vi "Deinitialize Robot.vi"(8 "error in":errorcluster, 11 "Gantry in":refnum<class "Gantry.lvclass">) -> (0 "error out":errorcluster, 3 "Gantry out":refnum<class "Gantry.lvclass">)   [LabVIEW 2026, in "Gantry.lvclass"]
uses:
  Gantry.lvclass
  <instrlib>/Aerotech Automation1/Aerotech Automation1.lvlib
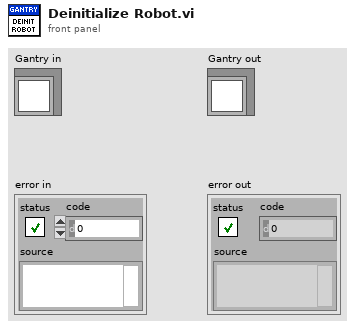
[diagram p1: front panel]
types:
  T1 = typedef "Virtual Modes.ctl" = enum16{"Nonvirtual", "Virtual"}
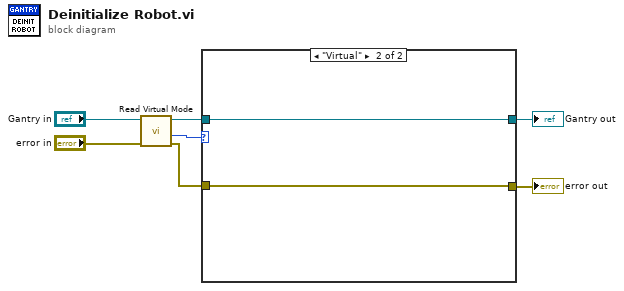
[diagram p0: block diagram]
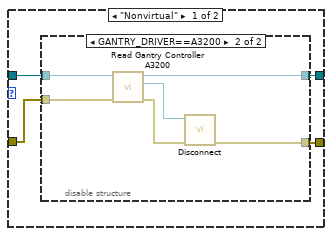
[diagram p2: hidden frame]
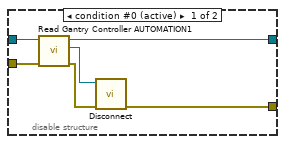
[diagram p3: hidden frame]
diagram:
  n1 = call-dynamic "Read Virtual Mode.vi"("error in (no error)"="error in", "Gantry in"="Gantry in") -> ("error out"=w3:errorcluster, "Virtual Mode"=w2:T1, "Gantry out"=w5:refnum<class "Gantry.lvclass">)  [unwired: 6 in, 1 out]
  n2 = case shown="\"Virtual\"" w2 {
    tunnel: [w9 w24] -> w7
    tunnel: w3 -> [w10 w24]
    tunnel: w5 -> [w11 w25]
    tunnel: [w8 w25] -> w1
    frame "Nonvirtual" {
      n3 = disable-structure shown="GANTRY_DRIVER==A3200" {
        disable-tunnel: w11 -> [w17 w21]
        disable-tunnel: w10 -> [w16 w20]
        disable-tunnel: [w13 w19] -> w9
        disable-tunnel: [w12 w18] -> w8
        frame condition #0 (active) {
          n4 = call "Read Gantry Controller AUTOMATION1.vi"("error in (no error)"=w16, "Gantry in"=w17) -> ("error out"=w15:errorcluster, "Controller AUTOMATION1"=w14:refnum<k24>, "Gantry out"=w12:refnum<class "Gantry.lvclass">)  [unwired: 7 in]
          n5 = call <instrlib>:"Disconnect.vi"("error in (no error)"=w15, "Controller Refnum in"=w14) -> ("error out"=w13:errorcluster)  [unwired: 9 in]
        }
        frame condition #1 {
          n6 = call "Read Gantry Controller A3200.vi"("error in (no error)"=w20, "Gantry in"=w21) -> ("error out"=w23:errorcluster, "A3200 controller out"=w22:refnum<k24>, "Gantry out"=w18:refnum<class "Gantry.lvclass">)  [unwired: 7 in]
          n7 = call <instrlib>:"Disconnect.vi"("error in (no error)"=w23, "controller"=w22) -> ("error out"=w19:errorcluster)  [unwired: 9 in]
        }
      }
    }
    frame "Virtual" {
    }
  }
  "error out" <- w7
  "Gantry out" <- w1
